vi "Read Config.vi"(8 "error in (no error)":errorcluster, 11 "LiDAR in":refnum<class "LiDAR.lvclass">) -> (0 "error out":errorcluster, 2 "LiDAR":T1, 3 "LiDAR out":refnum<class "LiDAR.lvclass">)   [LabVIEW 2018, in "LiDAR.lvlib" / "LiDAR.lvclass"]
uses:
  LiDAR.lvclass
  PPLs/Configuration/Configuration.lvlibp/Configuration.lvclass
  LiDAR.lvclass/LiDAR.ctl
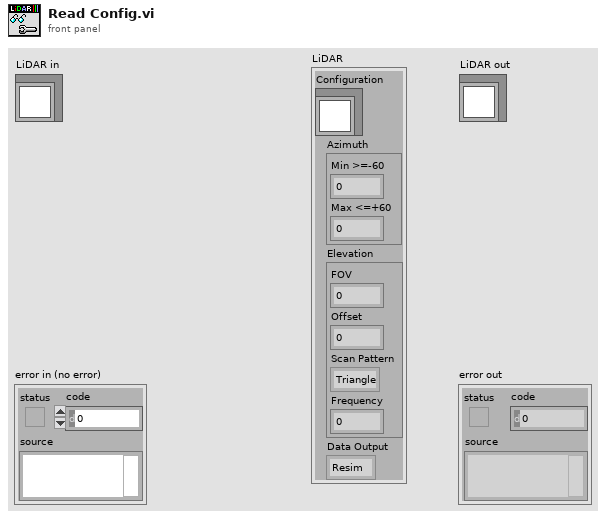
[diagram p1: front panel]
types:
  T1 = cluster{"Configuration":refnum<class "Configuration.lvclass">, "Azimuth":cluster{"Min >=-60":dbl, "Max <=+60 ":dbl}, "Elevation":cluster{"FOV":dbl, "Offset":dbl, "Scan Pattern":enum16{"Triangle", "Snap"}, "Frequency":dbl}, "Data Output":enum16{"Resim", "Point Cloud"}}
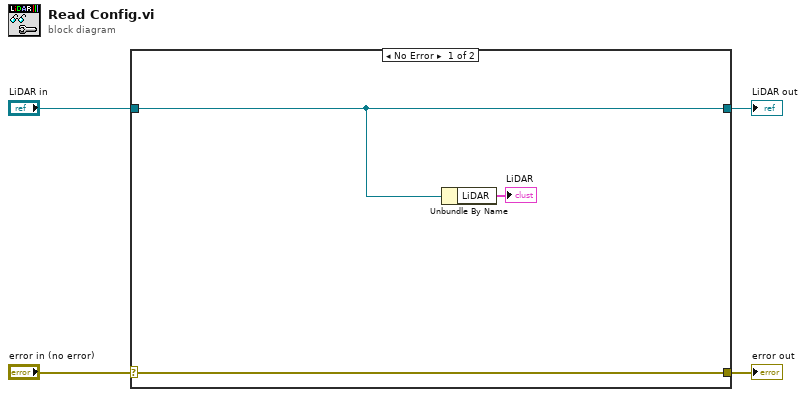
[diagram p0: block diagram]
diagram:
  n1 = case shown="No Error" "error in (no error)" {
    selector: "error in (no error)" -> [w7 w9]
    tunnel: [w7 w9] -> w3
    tunnel: [w6 w8] -> w1
    tunnel: "LiDAR in" -> [w6 w8]
    frame No Error {
      n2 = Unbundle By Name(w6) -> ("LiDAR"=→"LiDAR":T1)
    }
    frame Error {
    }
  }
  "error out" <- w3
  "LiDAR out" <- w1
